vi "CloseModuleManager.vi"(8 "error in (no error)":errorcluster, 11 "Sensor Engine Datas in":T1[](array[typedef])) -> (0 "error out":errorcluster, 3 "Sensor Engine Datas out":T1[](array[typedef]))   [LabVIEW 2023, in "MM.lvlib"]
uses:
  MM.lvlib
  Sensor Engine Data.ctl
  DataContainer/DataContainer.lvclass
  Shared/Protocol.ctl
  Shared/Vires VTD Shared.lvlib
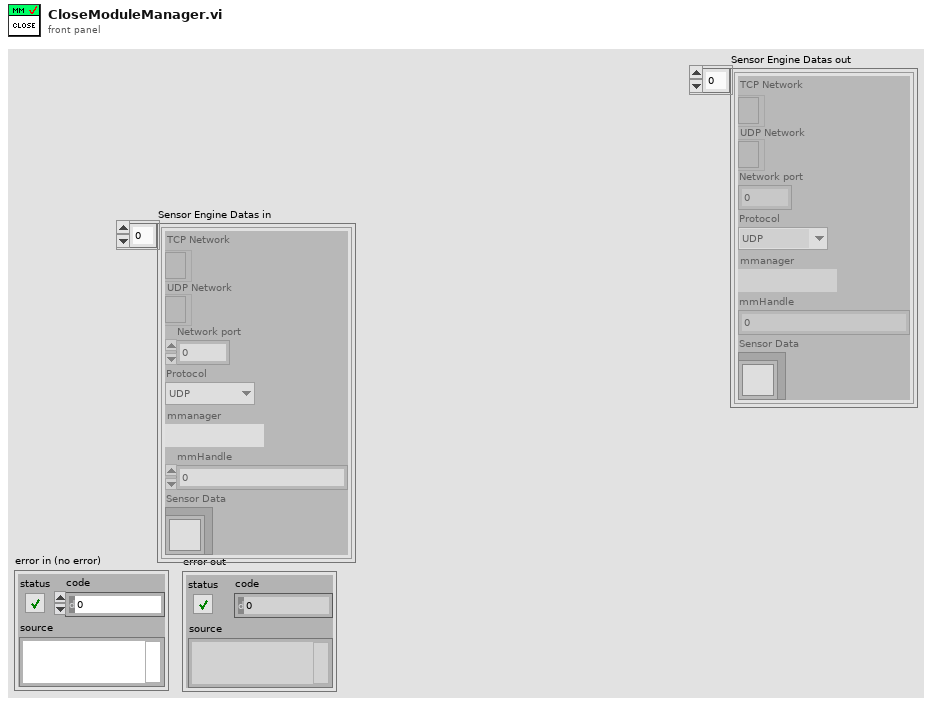
[diagram p1: front panel]
types:
  T1 = typedef "MM.lvlib/Sensor Engine Data.ctl" = cluster{"TCP Network":refnum<k5>, "UDP Network":refnum<k16>, "Network port":i32, "Protocol":T2, "mmanager":path, "mmHandle":u64, "Sensor Data":refnum<class "DataContainer.lvclass">}
  T2 = typedef "Vires VTD Shared.lvlib/Protocol.ctl" = enum16{"UDP", "TCP"}
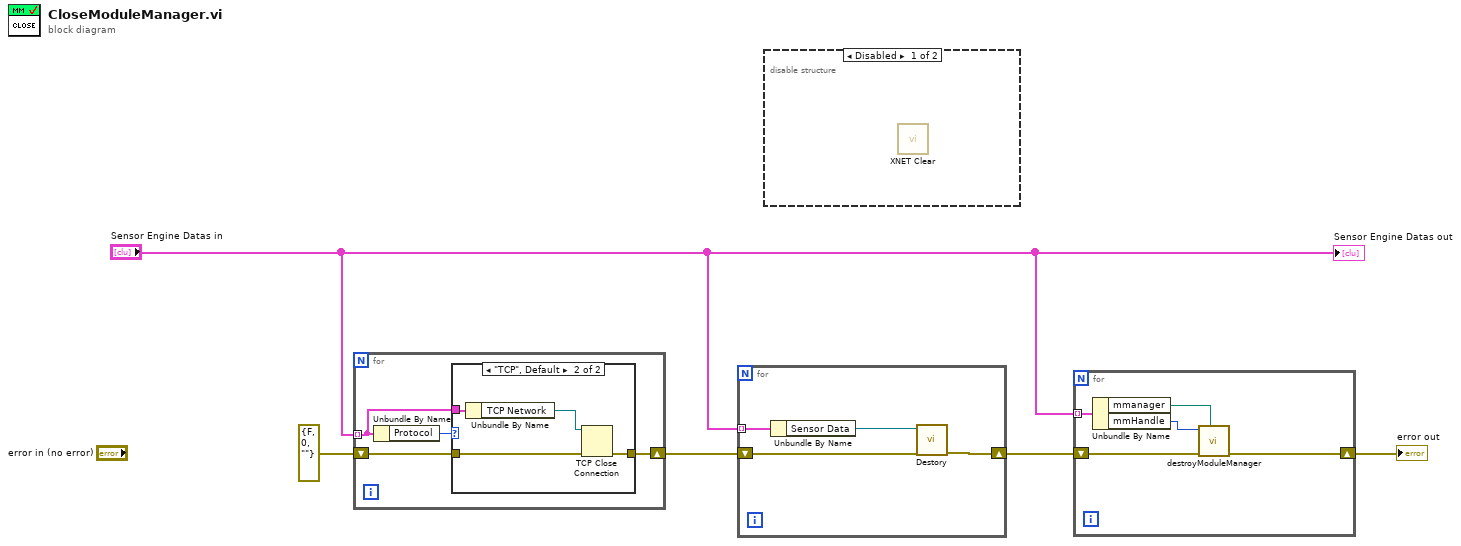
[diagram p0: block diagram]
diagram:
  n1 = for {
    shift-right: [w8] -> w5
    shift-left: errorcluster {"status"=FALSE, "code"=0, "source"=""} ("error out") -> [w9]
    tunnel: "Sensor Engine Datas in" -> [w6] mode=indexing
    n2 = Unbundle By Name(w6) -> ("Protocol"=w7:T2)
    n3 = case shown="\"TCP\", Default" w7 {
      tunnel: w9 -> [w10 w14]
      tunnel: [w10 w13] -> w8
      tunnel: w6 -> [_ w12]
      frame "UDP" {
      }
      frame "TCP", Default {
        n4 = Unbundle By Name(w12) -> ("TCP Network"=w11:refnum<k5>)
        n5 = TCP Close Connection(connection ID=w11, error in (no error)=w14) -> (error out=w13:errorcluster)  [unwired: 1 in, 1 out]
      }
    }
  }
  n6 = for {
    shift-right: [w17] -> w2
    shift-left: w5 -> [w18]
    tunnel: "Sensor Engine Datas in" -> [w16] mode=indexing
    n7 = Unbundle By Name(w16) -> ("Sensor Data"=w15:refnum<class "DataContainer.lvclass">)
    n8 = call-dynamic "Destory.vi"("error in (no error)"=w18, "DataContainer in"=w15) -> ("error out"=w17:errorcluster)  [unwired: 8 in, 1 out]
  }
  n9 = disable-structure shown="Disabled" {
    frame Disabled {
      n10 = call <vilib>:"XNET Clear.vi"() -> ()  [unwired: 15 in, 1 out]
    }
    frame Enabled {
    }
  }
  n11 = for {
    tunnel: "Sensor Engine Datas in" -> [w23] mode=indexing
    shift-right: [w19] -> w1
    shift-left: w2 -> [w20]
    n12 = Unbundle By Name(w23) -> ("mmanager"=w22:path, "mmHandle"=w21:u64)
    n13 = call "destroyModuleManager.vi"("path in"=w22, "error in (no error)"=w20, "mmHandle"=w21) -> ("error out"=w19:errorcluster)  [unwired: 8 in]
  }
  "error out" <- w1
  "Sensor Engine Datas out" <- "Sensor Engine Datas in"
